vi "002_FlowChart.vi"(11 "Queue Ref":T1={"UI"=refnum, "Message"=refnum, "Data"=refnum, "Caller"=refnum, "Name"="000 Common", "Data Path"=path "", "Class Path"=path "", "SubPanel"=refnum, "Project Name"="", "MNT"="", "Title"="", "Data Source"=refnum, "Queue List"={}, "VI"=refnum, "UE"=refnum}) -> ()   [LabVIEW 2020]
doc: "0014_XAJD_1500W-Flow Chart"
uses:
  Alin/QMH/000 Module Data Type.ctl
  Alin/QMH/Queue Message.ctl
  <vilib>/Utility/miscctls.llb/LVPoint32TypeDef.ctl
  a1345304-ed38-41b0-8c79-7ce0969963d6.vi
  <vilib>/Utility/file.llb/Read Delimited Spreadsheet (string).vi
  <vilib>/Utility/file.llb/Write Delimited Spreadsheet (string).vi
panel:
  out "QN":i32
  in  "ShowLable":bool
  in  "Chart Select":u16(ring) items=["0014_XAJD_1500W.vi", "0014_XAJD_1500W_1.vi"]
  in  "Panel Show":bool
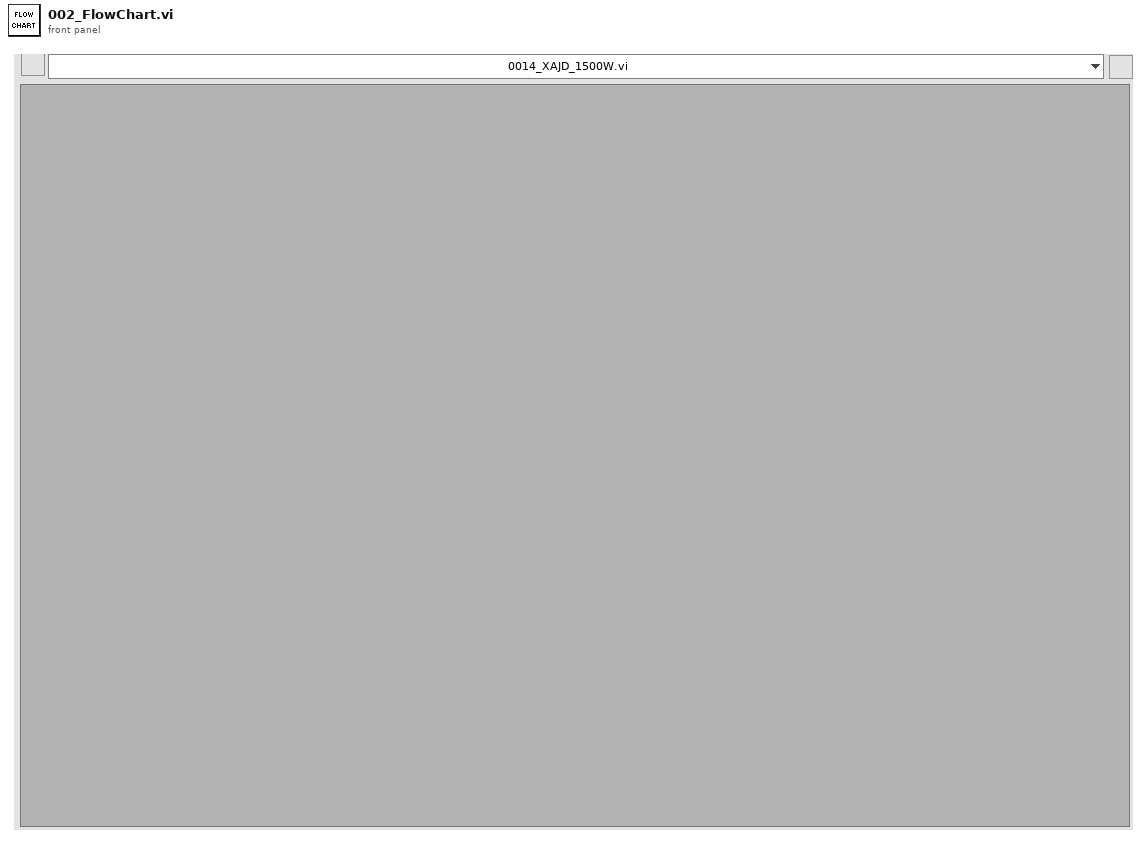
[diagram p1: front panel]
types:
  T1 = typedef "000 Module Data Type.ctl" = cluster{"UI":refnum<queue>, "Message":refnum<queue>, "Data":refnum<queue>, "Caller":refnum<queue>, "Name":string, "Data Path":path, "Class Path":path, "SubPanel":refnum<vi>, "Project Name":string, "MNT":string, "Title":string, "Data Source":refnum<queue>, "Queue List":map{string, refnum<queue>}, "VI":refnum<vi>, "UE":refnum<user-event>}
  T2 = enum32{"Invalid", "Standard", "Closed", "Hidden", "Minimized", "Maximized"}
  T3 = cluster{"Queue Ref":T1, "Flow Chart":refnum<vi>, "Controls":refnum<vi>[], "Delay":cluster{"Count Time(ms)":u32, "Delay Time(ms)":u32, "Next":string}}
  T4 = typedef "SDQ Data Type.ctl" = cluster{"CAN Length":string, "CAN Name":string, "CAN ID":string, "CAN Type":string, "Test Item":string, "Byte Order":string, "Instruction":string, "Control Type":string, "Group":string, "Offset":dbl, "Coefficient":dbl, "Write Enable":bool, "Lable Type":string, "Key?":string, "Set Value":string, "Upper":dbl, "Lower":dbl, "Unit":string, "Formula":string, "Test Item Type":string, "Length":i32, "Address":string, "Name":string, "Identifier":string, "Data Type":string, "Enumerate?":string, "Enumerate List":string, "Data":string, "Source":string}
  T5 = enum8{"Enabled", "Disabled", "Disabled and Grayed Out"}
  T6 = typedef "eventvkey.ctl" = enum16{"ASCII", "Enter", "Return", "Shift", "Ctrl", "Alt", "Cmd", "Opt", "Caps", "NumLock", "Clear", "Break", "Up", "Down", "Left", "Right", "Insert", "Delete", "Home", "End", "PageUp", "PageDown", "Escape", "Help", "Pause", "ScrollLock", "F1", "F2", "F3", "F4", "F5", "F6", "F7", "F8", "F9", "F10", "F11", "F12", "F13", "F14", "F15", "F16", "F17", "F18", "F19", "F20", "F21", "F22", "F23", "F24", "Play", "VolumeUp", "VolumeDown", "Mute", "Two Byte Char"}
  T7 = cluster{"Shift":bool, "Ctrl":bool, "Alt":bool, "Cmd":bool, "Opt":bool}
  T8 = typedef "LVPoint32TypeDef.ctl" = cluster{"Horizontal":i32, "Vertical":i32}
  T9 = cluster{"Queue List":map{string, refnum<queue>}, "SubPanel":refnum<vi>, "Active Panel":string, "Queue Ref":T1, "Project Name":string, "FlowChart":refnum<vi>, "Controls":refnum<vi>[]}
  T10 = typedef "LVBoundsTypeDef.ctl" = cluster{"Width":u32, "Height":u32}
  T11 = typedef "LVPointTypeDef.ctl" = cluster{"Horizontal":i16, "Vertical":i16}
  T12 = typedef "LVPositionTypeDef.ctl" = cluster{"Left":i32, "Top":i32}
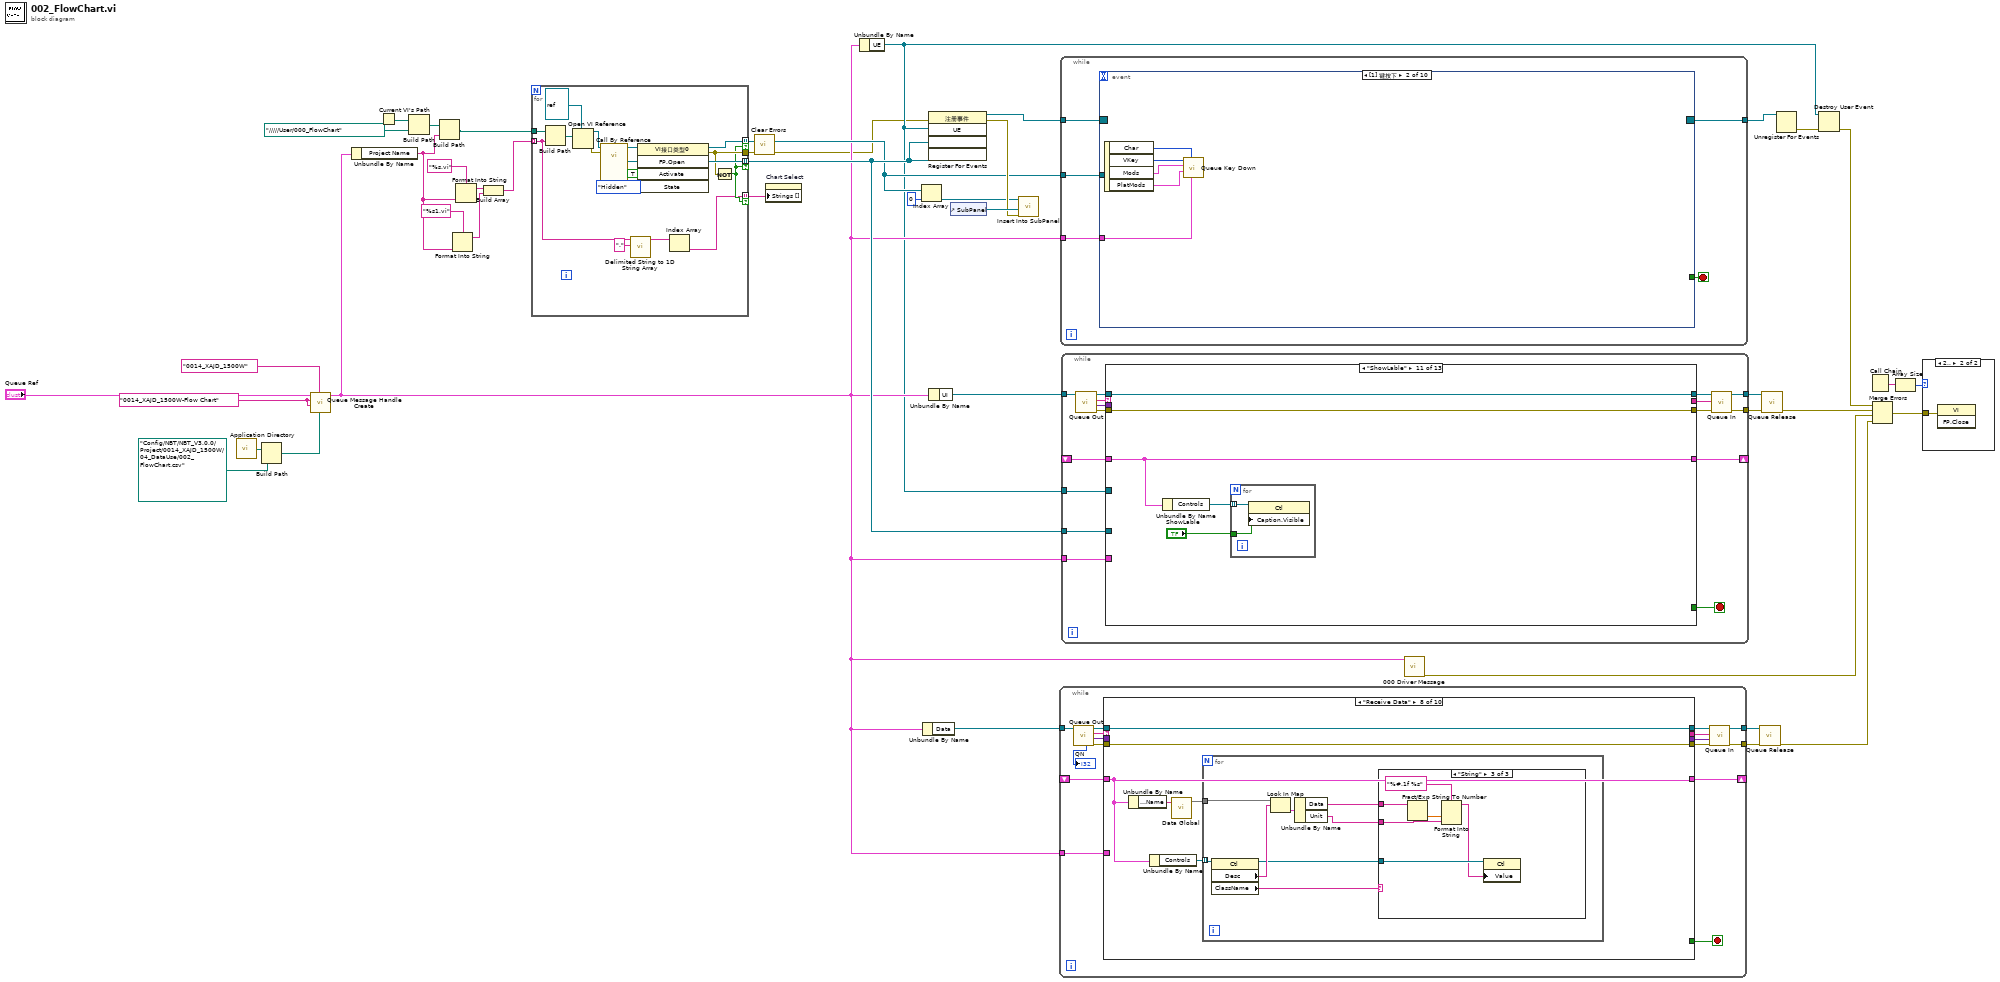
[diagram p0: block diagram]
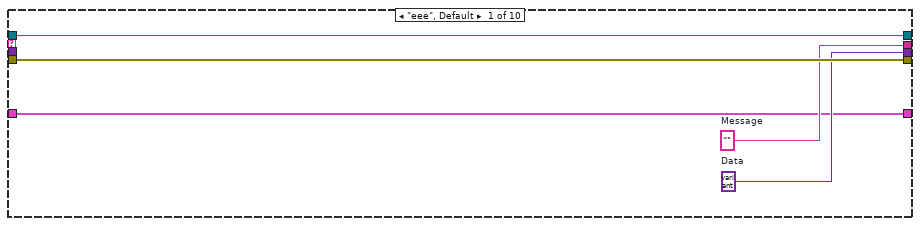
[diagram p2: hidden frame]
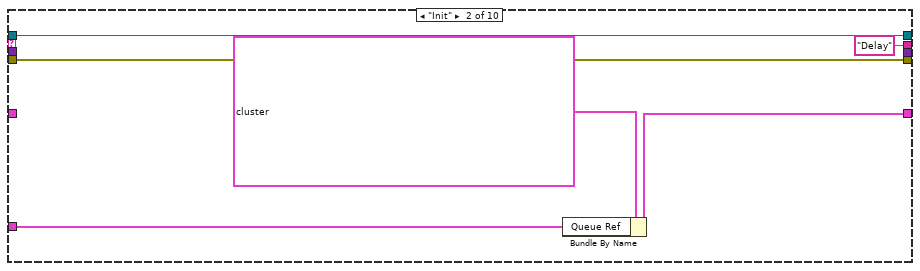
[diagram p3: hidden frame]
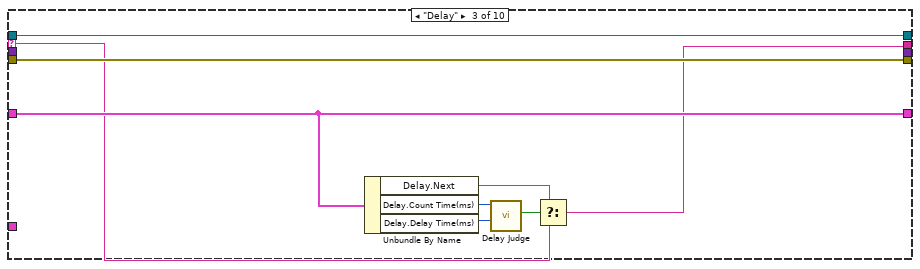
[diagram p4: hidden frame]
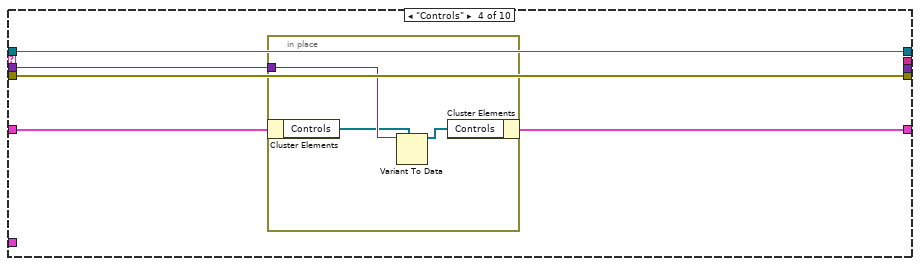
[diagram p5: hidden frame]
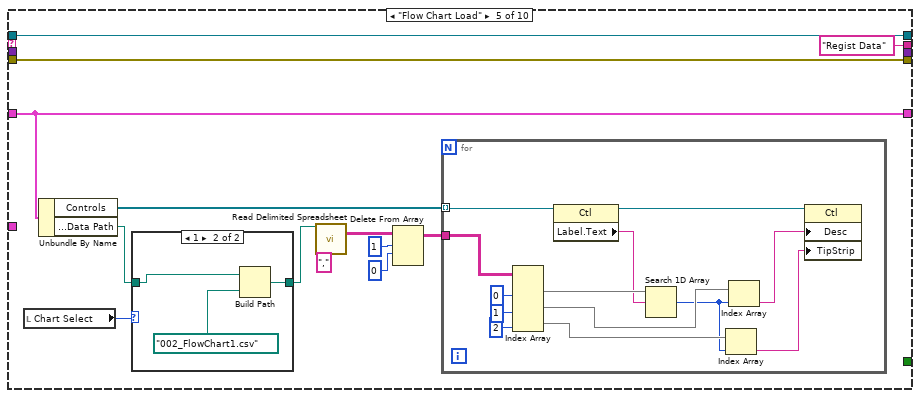
[diagram p6: hidden frame]
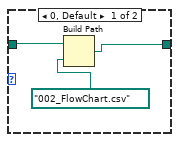
[diagram p7: hidden frame]
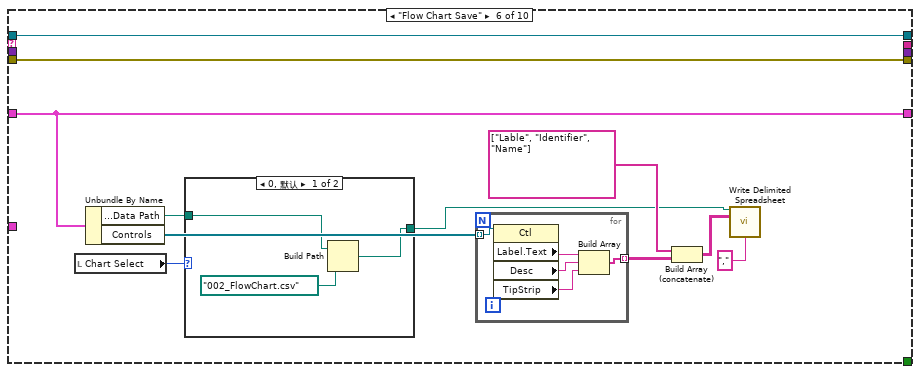
[diagram p8: hidden frame]
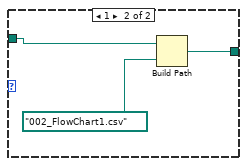
[diagram p9: hidden frame]
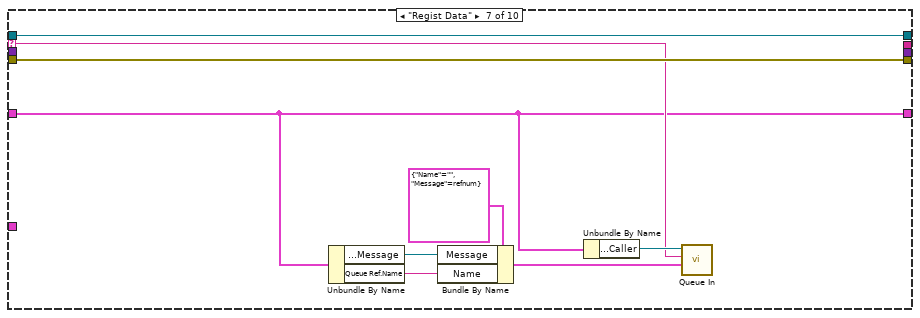
[diagram p10: hidden frame]
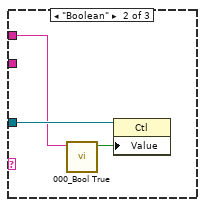
[diagram p12: hidden frame]
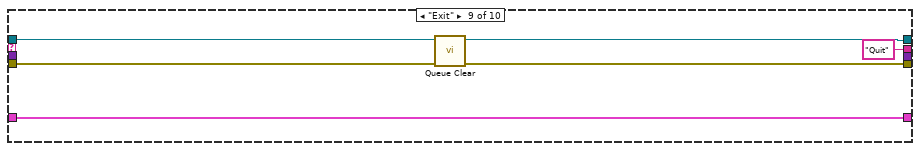
[diagram p13: hidden frame]
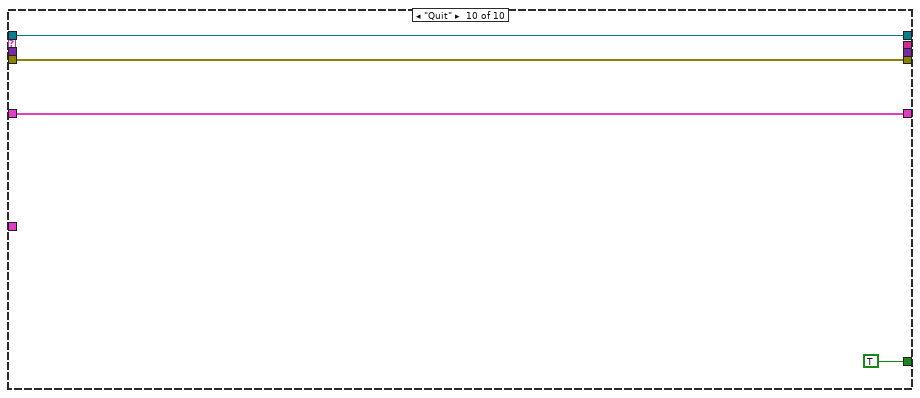
[diagram p14: hidden frame]
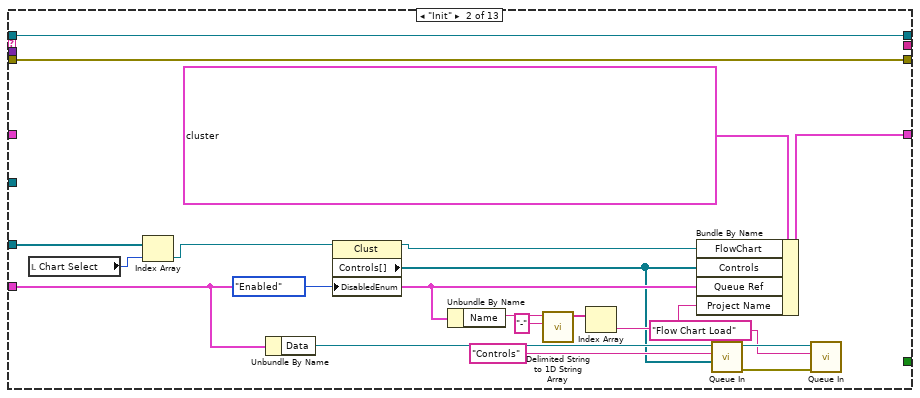
[diagram p17: hidden frame]
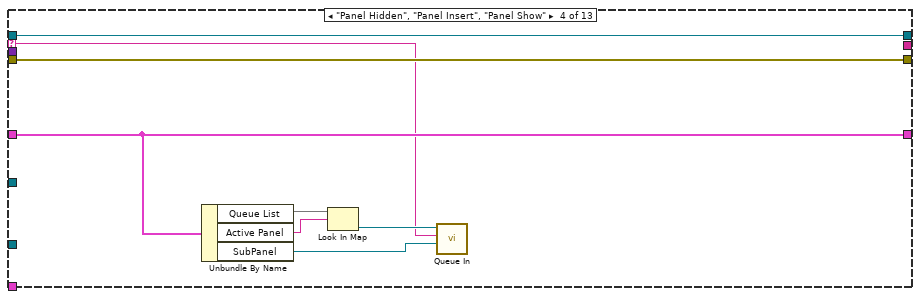
[diagram p19: hidden frame]
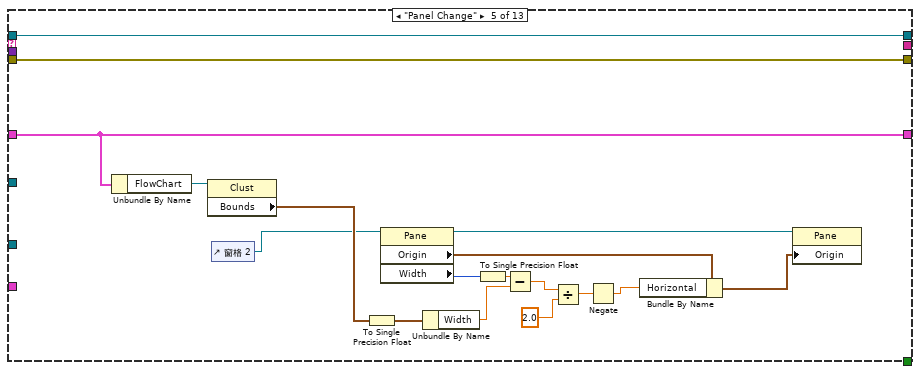
[diagram p20: hidden frame]
diagram:
  w6 = "0014_XAJD_1500W-Flow Chart" ("Name")
  n1 = call <vilib>:"Application Directory.vi"() -> ("Application Directory"=w9:path)
  n2 = Build Path(base path=w9, name or relative path=path "Config/NBT/NBT_V3.0.0/Project/0014_XAJD_1500W/04_DataUse/002_FlowChart.csv" ("名称或相对路径")) -> (appended path=w7:path)
  n3 = call "Queue Message Handle Create.vi"("Data Path"=w7, "Project Name"="0014_XAJD_1500W" ("Name"), "Name"=w6, "Title"=w6, "Queue Ref In"="Queue Ref") -> ("Queue Ref Out"=w3:T1)  [unwired: 5 in, 1 out]
  n4 = Unbundle By Name(w3) -> ("Project Name"=w12:string)
  n5 = Current VI's Path() -> (path=w27:path)
  n6 = Build Path(base path=w27, name or relative path=path "../../../../../User/000_FlowChart" ("名称或相对路径")) -> (appended path=w25:path)
  n7 = Build Path(base path=w25, name or relative path=w12) -> (appended path=w19:path)
  n8 = Format Into String(format string="%s1.vi" ("格式字符串"), w12) -> (resulting string=w11:string)  [unwired: 2 in, 1 out]
  n9 = Format Into String(format string="%s.vi" ("格式字符串"), w12) -> (resulting string=w17:string)  [unwired: 2 in, 1 out]
  n10 = Build Array(w17, w11) -> (w10:string[])
  n11 = for {
    tunnel: [w49] -> w22
    tunnel: [w53] -> w14 mode=indexing if=w48
    tunnel: [w52] -> w21 mode=indexing if=w48
    tunnel: w19 -> [w51]
    tunnel: w10 -> [w47] mode=indexing
    tunnel: [w44] -> w4 mode=indexing if=w48
    n12 = Build Path(base path=w51, name or relative path=w47) -> (appended path=w50:path)
    n13 = Open VI Reference(type specifier VI Refnum (for type only)=refnum<vi> refnum ("类型说明符VI引用句柄（仅用于类型）"), vi path=w50) -> (vi reference=w58:refnum<vi>, error out=w59:errorcluster)  [unwired: 4 in]
    n14 = call-by-ref "?"(reference=w58, error in=w59) -> (reference out=w56:refnum<vi>, "Cluster"=w52:refnum<vi>)  [unwired: 11 in, 1 out]
    n15 = call <vilib>:"Delimited String to 1D String Array.vi"("delimiter"=".", "delimited string"=w47) -> ("string array"=w45:string[])  [unwired: 9 in]
    n16 = invoke class="VI接口类型0" method="FP.Open"(reference=w56, "Activate"=TRUE ("激活？"), "State"=T2."Hidden" ("状态")) -> (reference out=w53:refnum<vi>, error out=w49:errorcluster)  [unwired: 2 in, 3 out]
    n17 = Index Array(array=w45) -> (element=w44:string)  [unwired: 1 in]
    n18 = Not(x=w49) -> (.not. x?=w48:bool)
  }
  n19 = call <vilib>:"Clear Errors.vi"("error in (no error)"=w22) -> ("error out"=w1:errorcluster)  [unwired: 5 in, 1 out]
  n20 = property on="Chart Select" class="Ring (严格)"("Strings []"=w4) -> ()  [unwired: 2 in, 2 out]
  n21 = Unbundle By Name(w3) -> ("UE"=w2:refnum<user-event>)
  n22 = Index Array(array=w14, index=0 ("索引")) -> (element=w16:refnum<vi>)
  n23 = Unbundle By Name(w3) -> ("Data"=w41:refnum<queue>)
  n24 = register-events(error in=w1, w2, w21, w21) -> (reference out=w28:refnum<event-registration>, error out=w23:errorcluster)  [unwired: 1 in]
  n25 = Unbundle By Name(w3) -> ("UI"=w33:refnum<queue>)
  n26 = control-ref of="SubPanel"() -> (w24:refnum<vi>)
  n27 = call "Insert Into SubPanel.vi"("error in (no error)"=w23, "SubPanel Ref"=w24, "VI Ref In"=w16) -> ()  [unwired: 8 in, 1 out]
  n28 = while {
    tunnel: w41 -> [w71]
    tunnel: [w68] -> w39
    tunnel: [w67] -> w40
    shift-right: [w63] -> _
    shift-left: _ -> [w62]
    tunnel: w3 -> [w61]
    stop <- w75 stop-if-true
    n29 = call "Queue Out.vi"("Queue In"=w71) -> ("error out"=w74:errorcluster, "Data"=w72:variant, "Message"=w73:string, "Queue Out"=w70:refnum<queue>, "Queue NUmber"=→"QN":i32)  [unwired: 6 in]
    n30 = case shown="\"Receive Data\"" w73 {
      selector: w73 -> [_ _ w88 _ _ _ w162 _ _ _]
      tunnel: w70 -> [w80 w86 w95 w100 w116 w146 w166 w172 w194 w198]
      tunnel: w74 -> [w79 w85 w94 w99 w115 w145 w165 w171 w192 w199]
      tunnel: [w80 w86 w95 w100 w116 w146 w166 w172 w193 w198] -> w69
      tunnel: [w79 w85 w94 w99 w115 w145 w165 w171 w191 w199] -> w66
      tunnel: [w78 "Delay" ("Message") w87 _ "Regist Data" ("Message") _ _ _ "Quit" _] -> w65
      tunnel: [_ _ _ _ _ _ _ _ _ TRUE] -> w75
      tunnel: [w77 _ _ _ _ _ _ _ _ _] -> w64
      tunnel: w72 -> [_ _ _ w96 _ _ _ _ _ _]
      tunnel: [w76 w83 w89 w97 w114 w144 w159 w168 w190 w196] -> w63
      tunnel: w62 -> [w76 _ w89 w98 w114 w144 w159 w168 w190 w196]
      tunnel: w61 -> [_ w82 _ _ _ _ _ _ _ _]
      frame "eee", Default {
        w77 = variant  # Data
        w78 = ""  # Message
      }
      frame "Init" {
        n31 = Bundle By Name(cluster=T3 {"Queue Ref"={"UI"=refnum, "Message"=refnum, "Data"=refnum, "Caller"=refnum, "Name"="", "Data Path"=path "", "Class Path"=path "", "SubPanel"=refnum, "Project Name"="", "MNT"="", "Title"="", "Data Source"=refnum, "Queue List"={}, "VI"=refnum, "UE"=refnum}, "Flow Chart"=refnum, "Controls"=[], "Delay"={"Count Time(ms)"=250, "Delay Time(ms)"=250, "Next"="Receive Data,Delay"}}, "Queue Ref"=w82) -> (w83:T3)
      }
      frame "Delay" {
        n32 = Unbundle By Name(w89) -> ("Delay.Next"=w93:string, "Delay.Count Time(ms)"=w90:u32, "Delay.Delay Time(ms)"=w91:u32)
        n33 = call "Delay Judge.vi"("Delay Time(ms)"=w91, "Count Time(ms)"=w90) -> ("Time Out?"=w92:bool)  [unwired: 5 in, 4 out]
        n34 = Select(t=w93, s=w92, f=w88) -> (s? t:f=w87:string)
      }
      frame "Controls" {
        n35 = in-place {
          in-place-border: w96 -> [w103]
          n36 = in-place-cluster #1(w98) -> ("Controls"=w102:refnum<vi>[])
          n37 = Variant To Data(type=w102, Variant=w103) -> (data=w101:refnum<vi>[])  [unwired: 1 in, 1 out]
          n38 = in-place-cluster #1("Controls"=w101) -> (w97:T3)
        }
      }
      frame "Flow Chart Load" {
        n39 = local read "Chart Select"() -> (w106:u16)
        n40 = Unbundle By Name(w114) -> ("Controls"=w113:refnum<vi>[], "Queue Ref.Data Path"=w105:path)
        n41 = case shown="1" w106 {
          tunnel: w105 -> [w119 w120]
          tunnel: [w117 w121] -> w104
          frame 0, Default {
            n42 = Build Path(base path=w119, name or relative path=path "002_FlowChart.csv" ("名称或相对路径")) -> (appended path=w117:path)
          }
          frame 1 {
            n43 = Build Path(base path=w120, name or relative path=path "002_FlowChart1.csv" ("名称或相对路径")) -> (appended path=w121:path)
          }
        }
        n44 = call-poly <vilib>:"Read Delimited Spreadsheet.vi"("file path (dialog if empty)"=w104, "delimiter (\\t)"="," ("delimiter (\\t)")) -> ("all rows"=w111:string[][])  [unwired: 8 in, 5 out]
        n45 = Delete From Array(array=w111, length=1 ("长度"), index (row)=0 ("索引 (行)")) -> (array with subset deleted=w108:string[][])  [unwired: 1 in, 1 out]
        n46 = for {
          tunnel: w113 -> [w135] mode=indexing
          tunnel: w108 -> [w134]
          n47 = Index Array(array=w134, index (col) #1=0 ("禁用的索引 (列)"), index (col) #2=1 ("索引 (列)"), index (col) #3=2 ("索引 (列)")) -> (element #1=w131:string[], element #2=w129:string[], element #3=w125:string[])  [unwired: 3 in]
          n48 = property class="Ctl"(reference=w135) -> (reference out=w128:refnum<vi>, "Label.Text"=w130:string)  [unwired: 1 in, 1 out]
          n49 = Search 1D Array(1D array=w131, element=w130) -> (index of element=w124:i32)  [unwired: 1 in]
          n50 = Index Array(array=w125, index=w124) -> (element=w123:string)
          n51 = Index Array(array=w129, index=w124) -> (element=w127:string)
          n52 = property class="Ctl"(reference=w128, "Desc"=w127, "TipStrip"=w123) -> ()  [unwired: 1 in, 2 out]
        }
      }
      frame "Flow Chart Save" {
        n53 = local read "Chart Select"() -> (w138:u16)
        n54 = Unbundle By Name(w144) -> ("Queue Ref.Data Path"=w137:path, "Controls"=w143:refnum<vi>[])
        n55 = case shown="0, 默认" w138 {
          tunnel: w137 -> [w148 w152]
          tunnel: [w149 w150] -> w136
          frame 0, Default {
            n56 = Build Path(base path=w148, name or relative path=path "002_FlowChart.csv" ("名称或相对路径")) -> (appended path=w149:path)
          }
          frame 1 {
            n57 = Build Path(base path=w152, name or relative path=path "002_FlowChart1.csv" ("名称或相对路径")) -> (appended path=w150:path)
          }
        }
        n58 = for {
          tunnel: w143 -> [w157] mode=indexing
          tunnel: [w154] -> w141 mode=indexing
          n59 = property class="Ctl"(reference=w157) -> ("Label.Text"=w156:string, "Desc"=w155:string, "TipStrip"=w153:string)  [unwired: 1 in, 2 out]
          n60 = Build Array(w156, w155, w153) -> (w154:string[])
        }
        n61 = Build Array (concatenate)(string[] ["Lable", "Identifier", "Name"], w141) -> (w140:string[][])
        n62 = call-poly <vilib>:"Write Delimited Spreadsheet.vi"("file path (dialog if empty)"=w136, "2D data"=w140, "delimiter (\\t)"="," ("delimiter (\\t)")) -> ()  [unwired: 11 in, 2 out]
      }
      frame "Regist Data" {
        n63 = Unbundle By Name(w159) -> ("Queue Ref.Message"=w160:refnum<queue>, "Queue Ref.Name"=w158:string)
        n64 = Bundle By Name(cluster=cluster{"Name":string, "Message":refnum<queue>} {"Name"="", "Message"=refnum} ("输出簇"), "Message"=w160, "Name"=w158) -> (w161:cluster{"Name":string, "Message":refnum<queue>})
        n65 = Unbundle By Name(w159) -> ("Queue Ref.Caller"=w163:refnum<queue>)
        n66 = call "Queue In.vi"("Data"=w161, "Message"=w162, "Queue In"=w163) -> ()  [unwired: 7 in, 2 out]
      }
      frame "Receive Data" {
        n67 = Unbundle By Name(w168) -> ("Queue Ref.Name"=w169:string)
        n68 = Unbundle By Name(w168) -> ("Controls"=w170:refnum<vi>[])
        n69 = call "Data Global.vi"("Name"=w169) -> ("Data Out"=w167:map{string, T4})  [unwired: 7 in, 3 out]
        n70 = for {
          tunnel: w170 -> [w180] mode=indexing
          tunnel: w167 -> [w179]
          n71 = property class="Ctl"(reference=w180) -> (reference out=w175:refnum<vi>, "Desc"=w178:string, "ClassName"=w176:string)  [unwired: 1 in, 1 out]
          n72 = Look In Map(map=w179, key=w178) -> (value=w177:T4)  [unwired: 1 in, 1 out]
          n73 = Unbundle By Name(w177) -> ("Data"=w174:string, "Unit"=w173:string)
          n74 = case shown="\"String\"" w176 {
            tunnel: w175 -> [_ w183 w189]
            tunnel: w174 -> [_ w182 w186]
            tunnel: w173 -> [_ _ w184]
            frame "eee", Default {
            }
            frame "Boolean" {
              n75 = call "000_Bool True.vi"("Bool String"=w182) -> ("True"=w181:bool)  [unwired: 8 in, 2 out]
              n76 = property class="Ctl"(reference=w183, "Value"=w181) -> ()  [unwired: 1 in, 2 out]
            }
            frame "String" {
              n77 = Fract/Exp String To Number(string=w186) -> (number=w185:dbl)  [unwired: 3 in, 1 out]
              n78 = Format Into String(format string="%#.1f %s" ("格式字符串"), w185, w184) -> (resulting string=w187:string)  [unwired: 2 in, 1 out]
              n79 = property class="Ctl"(reference=w189, "Value"=w187) -> ()  [unwired: 1 in, 2 out]
            }
          }
        }
      }
      frame "Exit" {
        n80 = call "Queue Clear.vi"("error in (no error)"=w192, "Queue In"=w194) -> ("error out"=w191:errorcluster, "Queue Out"=w193:refnum<queue>)  [unwired: 8 in]
      }
      frame "Quit" {
      }
    }
    n81 = call "Queue In.vi"("error in (no error)"=w66, "Data"=w64, "Message"=w65, "Queue In"=w69) -> ("error out"=w67:errorcluster, "Queue Out"=w68:refnum<queue>)  [unwired: 6 in]
  }
  n82 = while {
    tunnel: w28 -> [w204]
    tunnel: [w202] -> w29
    tunnel: w3 -> [w201]
    tunnel: w14 -> [w200]
    stop <- w203 stop-if-true
    n83 = event shown="[1] 键按下" {
      selector: w204 -> [_ _ _ _ _ _ _ _ _ _]
      dyn-events: [_ _ _ _ _ _ _ _ _ _] -> w202
      timeout: _ -> [_ _ _ _ _ _ _ _ _ _]
      tunnel: [_ _ _ _ _ w243 _ _ _ _] -> w203
      tunnel: w201 -> [_ w208 w212 w218 w223 _ w247 w256 w264 w268]
      tunnel: w200 -> [_ _ _ _ _ _ _ w259 _ _]
      event Timeout {
        n84 = event-data() -> ()  [unwired: 1 in, 1 out]
      }
      event Key Down {
        n85 = event-data() -> ("Char"=w209:i16, "VKey"=w207:T6, "Mods"=w206:cluster{"Num Pad":bool, "Menu Key":bool}, "PlatMods"=w205:T7)  [unwired: 1 in]
        n86 = call "Queue Key Down.vi"("Queue Ref Out"=w208, "C"=w209, "Platform Key"=w205, "Group Key"=w206, "V Key"=w207) -> ()  [unwired: 6 in, 1 out]
      }
      event Panel Resize {
        n87 = event-data() -> ()  [unwired: 1 in, 1 out]
        n88 = Unbundle By Name(w212) -> ("Message"=w211:refnum<queue>)
        n89 = call "Queue In.vi"("Message"="Panel Change", "Queue In"=w211) -> ()  [unwired: 8 in, 2 out]
      }
      event Value Change {
        n90 = event-data() -> ("NewVal"=w217:variant, "OldVal"=w216:variant)  [unwired: 1 in]
        n91 = Unbundle By Name(w218) -> ("UI"=w215:refnum<queue>)
        n92 = call "FlowChart String Analize.vi"("Old Value"=w216, "New Value"=w217) -> ("Data"=w214:cluster{"Index":i32, "Data":variant})  [unwired: 7 in, 2 out]
        n93 = call "Queue In.vi"("Data"=w214, "Message"="Write Prepare", "Queue In"=w215) -> ()  [unwired: 7 in, 2 out]
      }
      event Mouse Down {
        n94 = event-data() -> ("CtlRef"=w220:refnum<vi>, "PlatMods.Shift"=w221:bool, "Coords"=w219:T8, "PlatMods.Alt"=w224:bool, "Mods.Double Click"=w225:bool)  [unwired: 1 in]
        n95 = Unbundle By Name(w223) -> ("UI"=w222:refnum<queue>)
        n96 = case shown="真" w225 {
          tunnel: w224 -> [_ w230]
          tunnel: w222 -> [_ w229]
          tunnel: w221 -> [_ w228]
          tunnel: w220 -> [_ w227]
          tunnel: w219 -> [_ w226]
          frame False {
          }
          frame True {
            n97 = case shown="真" w230 {
              tunnel: w229 -> [_ w242]
              tunnel: w228 -> [w232 _]
              tunnel: w227 -> [w231 _]
              tunnel: w226 -> [_ w240]
              frame False {
                n98 = case shown="真" w232 {
                  tunnel: w231 -> [_ w233]
                  frame False {
                  }
                  frame True {
                    n99 = property class="Clust"(reference=w233) -> (reference out=w235:refnum<vi>, "DisabledEnum"=w234:T5)  [unwired: 1 in, 1 out]
                    n100 = case shown="\"Enabled\", 默认" w234 {
                      tunnel: [T5."Disabled and Grayed Out" ("禁用") T5."Disabled and Grayed Out" ("禁用") T5."Enabled" ("禁用")] -> w236
                      frame "Enabled", Default {
                      }
                      frame "Disabled" {
                      }
                      frame "Disabled and Grayed Out" {
                      }
                    }
                    n101 = property class="Clust"(reference=w235, "DisabledEnum"=w236) -> ()  [unwired: 1 in, 2 out]
                  }
                }
              }
              frame True {
                n102 = call "Queue In.vi"("Data"=w240, "Message"="Show Data Source", "Queue In"=w242) -> ()  [unwired: 7 in, 2 out]
              }
            }
          }
        }
      }
      event User Event {
        n103 = event-data() -> ("Message"=w245:string)  [unwired: 1 in]
        n104 = Equal?(x=w245, y="Exit") -> (x = y?=w243:bool)
      }
      event Panel Close? {
        n105 = event-data() -> ()  [unwired: 1 in, 1 out]
        n106 = Unbundle By Name(w247) -> ("Message"=w246:refnum<queue>)
        n107 = Call Chain() -> (call chain=w250:string[])
        n108 = Array Size(array=w250) -> (size(s)=w249:i32)
        n109 = case shown="0, 默认" w249 {
          tunnel: ["Exit Prepare" ("Message") "Panel Hidden" ("Message")] -> w248
          frame 0, Default {
          }
          frame 2.. {
          }
        }
        n110 = call "Queue In.vi"("Message"=w248, "Queue In"=w246) -> ()  [unwired: 8 in, 2 out]
        n111 = event-data("Discard?"=TRUE ("放弃？")) -> ()  [unwired: 1 in, 1 out]
      }
      event "Chart Select": Value Change {
        n112 = event-data() -> ()  [unwired: 1 in, 1 out]
        n113 = Unbundle By Name(w256) -> ("UI"=w255:refnum<queue>)
        n114 = call "Queue In.vi"("Message"="Init", "Queue In"=w255) -> ()  [unwired: 8 in, 2 out]
        n115 = control-ref of="SubPanel"() -> (w260:refnum<vi>)
        n116 = Index Array(array=w259, index="Chart Select") -> (element=w257:refnum<vi>)
        n117 = call "Insert Into SubPanel.vi"("SubPanel Ref"=w260, "VI Ref In"=w257) -> ()  [unwired: 9 in, 1 out]
      }
      event "Panel Show": Value Change {
        n118 = event-data() -> ("CtlRef"=w262:refnum<vi>)  [unwired: 1 in]
        n119 = Unbundle By Name(w264) -> ("Message"=w263:refnum<queue>)
        n120 = property class="Bool"(reference=w262) -> ("Label.Text"=w261:string)  [unwired: 1 in, 2 out]
        n121 = call "Queue In.vi"("Message"=w261, "Queue In"=w263) -> ()  [unwired: 8 in, 2 out]
      }
      event "ShowLable": Value Change {
        n122 = event-data() -> ("CtlRef"=w266:refnum<vi>)  [unwired: 1 in]
        n123 = Unbundle By Name(w268) -> ("UI"=w267:refnum<queue>)
        n124 = property class="Bool (严格)"(reference=w266) -> ("Label.Text"=w265:string)  [unwired: 1 in, 2 out]
        n125 = call "Queue In.vi"("Message"=w265, "Queue In"=w267) -> ()  [unwired: 8 in, 2 out]
      }
    }
  }
  n126 = while {
    tunnel: w33 -> [w279]
    tunnel: [w276] -> w31
    tunnel: [w275] -> w32
    tunnel: w2 -> [w283]
    tunnel: w3 -> [w272]
    shift-right: [w271] -> _
    shift-left: _ -> [w270]
    tunnel: w21 -> [w269]
    stop <- w284 stop-if-true
    n127 = call "Queue Out.vi"("Queue In"=w279) -> ("error out"=w282:errorcluster, "Data"=w280:variant, "Message"=w281:string, "Queue Out"=w278:refnum<queue>)  [unwired: 6 in, 1 out]
    n128 = case shown="\"ShowLable\"" w281 {
      selector: w281 -> [_ _ _ w313 _ _ w346 _ _ _ _ w433 _]
      tunnel: w278 -> [w287 w307 w310 w318 w335 w340 w350 w353 w363 w409 w428 w440 w447]
      tunnel: w282 -> [w286 w306 w309 w317 w334 w339 w349 w352 w362 w408 w427 w438 w448]
      tunnel: [w287 w307 w310 w318 w335 w340 w350 w353 w363 w409 w428 w439 w447] -> w277
      tunnel: [w286 w306 w309 w317 w334 w339 w349 w352 w362 w408 w427 w437 w448] -> w274
      tunnel: [_ _ _ _ _ _ _ _ _ _ _ "Quit" _] -> w273
      tunnel: [_ _ _ _ _ _ _ _ _ _ _ _ TRUE] -> w284
      tunnel: w283 -> [_ _ _ _ _ _ _ _ _ _ _ _ _]
      tunnel: w280 -> [_ _ _ _ _ w336 _ _ w360 w406 _ _ _]
      tunnel: w272 -> [_ w294 _ _ _ _ w348 _ _ _ _ _ _]
      tunnel: [w285 w304 w308 w316 w333 w337 w345 w351 w354 w405 w426 w432 w445] -> w271
      tunnel: w270 -> [w285 _ w308 w316 w333 w338 w345 w351 w355 w405 w426 w432 w445]
      tunnel: w269 -> [_ w297 _ _ _ _ _ _ _ _ _ _ _]
      frame "eee", Default {
      }
      frame "Init" {
        n129 = local read "Chart Select"() -> (w296:u16)
        n130 = Index Array(array=w297, index=w296) -> (element=w295:refnum<vi>)
        n131 = Unbundle By Name(w294) -> ("Data"=w293:refnum<queue>)
        n132 = property class="Clust"(reference=w295, "DisabledEnum"=T5."Enabled" ("禁用")) -> (reference out=w298:refnum<vi>, "Controls[]"=w291:refnum<vi>[])  [unwired: 1 in, 1 out]
        n133 = Unbundle By Name(w294) -> ("Name"=w303:string)
        n134 = call <vilib>:"Delimited String to 1D String Array.vi"("delimiter"="-", "delimited string"=w303) -> ("string array"=w301:string[])  [unwired: 9 in]
        n135 = Index Array(array=w301) -> (element=w300:string)  [unwired: 1 in]
        n136 = Bundle By Name(cluster=T9 {"Queue List"={}, "SubPanel"=refnum, "Active Panel"="", "Queue Ref"={"UI"=refnum, "Message"=refnum, "Data"=refnum, "Caller"=refnum, "Name"="", "Data Path"=path "", "Class Path"=path "", "SubPanel"=refnum, "Project Name"="", "MNT"="", "Title"="", "Data Source"=refnum, "Queue List"={}, "VI"=refnum, "UE"=refnum}, "Project Name"="", "FlowChart"=refnum, "Controls"=[]}, "FlowChart"=w298, "Controls"=w291, "Queue Ref"=w294, "Project Name"=w300) -> (w304:T9)
        n137 = call "Queue In.vi"("Data"=w291, "Message"="Controls", "Queue In"=w293) -> ("error out"=w290:errorcluster, "Queue Out"=w289:refnum<queue>)  [unwired: 7 in]
        n138 = call "Queue In.vi"("error in (no error)"=w290, "Message"="Flow Chart Load", "Queue In"=w289) -> ()  [unwired: 7 in, 2 out]
      }
      frame "====System====" {
      }
      frame "Panel Hidden", "Panel Insert", "Panel Show" {
        n139 = Unbundle By Name(w316) -> ("Queue List"=w315:map{string, refnum<queue>}, "Active Panel"=w312:string, "SubPanel"=w311:refnum<vi>)
        n140 = Look In Map(map=w315, key=w312) -> (value=w314:refnum<queue>)  [unwired: 1 in, 1 out]
        n141 = call "Queue In.vi"("Data"=w311, "Message"=w313, "Queue In"=w314) -> ()  [unwired: 7 in, 2 out]
      }
      frame "Panel Change" {
        n142 = Unbundle By Name(w333) -> ("FlowChart"=w331:refnum<vi>)
        n143 = property class="Clust"(reference=w331) -> ("Bounds"=w332:T10)  [unwired: 1 in, 2 out]
        n144 = control-ref of="窗格 2"() -> (w319:refnum<vi>)
        n145 = To Single Precision Float(number=w332) -> (single precision float=w324:cluster{"Width":sgl, "Height":sgl})
        n146 = property class="Pane"(reference=w319) -> (reference out=w326:refnum<vi>, "Origin"=w322:T11, "Width"=w330:u32)  [unwired: 1 in, 1 out]
        n147 = Unbundle By Name(w324) -> ("Width"=w323:sgl)
        n148 = To Single Precision Float(number=w330) -> (single precision float=w325:sgl)
        n149 = Subtract(x=w325, y=w323) -> (x-y=w329:sgl)
        n150 = Divide(x=w329, y=sgl 2.0) -> (x/y=w327:sgl)
        n151 = Negate(x=w327) -> (-x=w321:sgl)
        n152 = Bundle By Name(cluster=w322, "Horizontal"=w321) -> (w320:T11)
        n153 = property class="Pane"(reference=w326, "Origin"=w320) -> ()  [unwired: 1 in, 2 out]
      }
      frame "Send Client Refer" {
        n154 = in-place {
          in-place-border: w336 -> [w342]
          n155 = in-place-cluster #2(w338) -> ("Queue List"=w341:map{string, refnum<queue>})
          n156 = Variant To Data(type=w341, Variant=w342) -> (data=w343:map{string, refnum<queue>})  [unwired: 1 in, 1 out]
          n157 = in-place-cluster #2("Queue List"=w343) -> (w337:T9)
        }
      }
      frame "Client Delete", "Client Launch" {
        n158 = Unbundle By Name(w348) -> ("Message"=w347:refnum<queue>)
        n159 = Unbundle By Name(w345) -> ("Active Panel"=w344:string)
        n160 = call "Queue In.vi"("Data"=w344, "Message"=w346, "Queue In"=w347) -> ()  [unwired: 7 in, 2 out]
      }
      frame "====User====" {
      }
      frame "Show Data Source" {
        n161 = Unbundle By Name(w355) -> ("FlowChart"=w359:refnum<vi>)
        n162 = Variant To Data(type=T8 {"Horizontal"=0, "Vertical"=0} ("坐标"), Variant=w360) -> (data=w356:T8)  [unwired: 1 in, 1 out]
        n163 = property class="Clust"(reference=w359) -> ("DisabledEnum"=w358:T5, "Controls[]"=w357:refnum<vi>[])  [unwired: 1 in, 2 out]
        n164 = case shown="\"Disabled and Grayed Out\"" w358 {
          tunnel: w357 -> [_ w368]
          tunnel: w356 -> [_ w367]
          tunnel: w355 -> [w364 w366]
          tunnel: [w364 w365] -> w354
          frame "Enabled", Default {
          }
          frame "Disabled and Grayed Out" {
            n165 = for {
              tunnel: w368 -> [w379] mode=indexing
              tunnel: w367 -> [w372]
              shift-right: [w371] -> w365
              shift-left: w366 -> [w370]
              stop <- w373 stop-if-true
              n166 = property class="Ctl"(reference=w379) -> (reference out=w369:refnum<vi>, "Bounds"=w375:T10, "Position"=w374:T12)  [unwired: 1 in, 1 out]
              n167 = Add(x=w375, y=w374) -> (x+y=w378:T10)
              n168 = In Range and Coerce(upper limit=w378, x=w372, lower limit=w374) -> (In Range?=w377:cluster{"Width":bool, "Height":bool})  [unwired: 1 out]
              n169 = Cluster To Array(cluster=w377) -> (array=w376:bool[])
              n170 = And Array Elements(Boolean array=w376) -> (logical AND=w373:bool)
              n171 = case shown="真" w373 {
                tunnel: [w380 w383] -> w371
                tunnel: w370 -> [w380 w383]
                tunnel: w369 -> [_ w389]
                frame False {
                }
                frame True {
                  n172 = Unbundle By Name(w383) -> ("Queue Ref.Data"=w381:refnum<queue>, "Queue Ref.Name"=w382:string)
                  n173 = property class="Ctl"(reference=w389) -> (reference out=w387:refnum<vi>, "Desc"=w388:string)  [unwired: 1 in, 1 out]
                  n174 = call "FlowChart Edit.vi"("Name"=w382, "Identifier In"=w388) -> ("OK？"=w386:bool, "Tips"=w384:string, "Identifier Out"=w385:string)  [unwired: 6 in, 1 out]
                  n175 = case shown="真" w386 {
                    tunnel: w387 -> [_ w394]
                    tunnel: w385 -> [_ w393]
                    tunnel: w384 -> [_ w392]
                    tunnel: w381 -> [_ w391]
                    frame False {
                    }
                    frame True {
                      n176 = property class="Ctl"(reference=w394, "Desc"=w393, "TipStrip"=w392) -> ()  [unwired: 1 in, 2 out]
                      n177 = call "Queue In.vi"("Message"="Flow Chart Save", "Queue In"=w391) -> ()  [unwired: 8 in, 2 out]
                    }
                  }
                }
              }
            }
          }
        }
      }
      frame "Write Prepare" {
        n178 = Unbundle By Name(w405) -> ("Queue Ref.Caller"=w395:refnum<queue>, "Controls"=w404:refnum<vi>[])
        n179 = Variant To Data(type=cluster{i32, "Value":string} {0, "Value"=""}, Variant=w406) -> (data=w407:cluster{i32, "Value":string})  [unwired: 1 in, 1 out]
        n180 = Unbundle(w407) -> (w402:i32, "Value"=w398:string)
        n181 = Index Array(array=w404, index=w402) -> (element=w403:refnum<vi>)
        n182 = Equal?(x=w398, y="1") -> (x = y?=w396:bool)
        n183 = property class="Ctl"(reference=w403) -> ("TipStrip"=w401:string, "Desc"=w400:string)  [unwired: 1 in, 2 out]
        n184 = case shown="\"eee\", 默认" w400 {
          selector: w400 -> [w411 _]
          tunnel: w401 -> [w414 _]
          tunnel: w396 -> [w410 _]
          tunnel: w395 -> [w412 _]
          frame "eee", Default {
            n185 = Select(t="打开", s=w410, f="关闭") -> (s? t:f=w415:string)
            n186 = Format Into String(format string="确定%s%s?" ("消息"), w415, w414) -> (resulting string=w418:string)  [unwired: 2 in, 1 out]
            n187 = Two Button Dialog(message=w418) -> (T button?=w413:bool)  [unwired: 2 in]
            n188 = case shown="真" w413 {
              tunnel: w412 -> [_ w423]
              tunnel: w411 -> [_ w422]
              tunnel: w410 -> [_ w421]
              frame False {
              }
              frame True {
                n189 = call "000_Bool True.vi"("Value"=w421) -> ("String Out"=w420:string)  [unwired: 8 in, 2 out]
                n190 = call "000_Source Write.vim"("Data"=w420, "Name"=w422, "Queue In"=w423) -> ()  [unwired: 6 in, 3 out]
              }
            }
          }
          frame "" {
          }
        }
      }
      frame "ShowLable" {
        n191 = Unbundle By Name(w426) -> ("Controls"=w425:refnum<vi>[])
        n192 = for {
          tunnel: w425 -> [w430] mode=indexing
          tunnel: "ShowLable" -> [w429]
          n193 = property class="Ctl"(reference=w430, "Caption.Visible"=w429) -> ()  [unwired: 1 in, 2 out]
        }
      }
      frame "Exit" {
        n194 = Unbundle By Name(w432) -> ("Queue Ref.UE"=w431:refnum<user-event>, "Queue Ref.Message"=w436:refnum<queue>, "Queue Ref.Data"=w435:refnum<queue>)
        n195 = Build Array(w436, w435) -> (w434:refnum<queue>[])
        n196 = for {
          tunnel: w434 -> [w444] mode=indexing
          tunnel: w433 -> [w443]
          n197 = call "Queue In.vi"("First"=TRUE, "Message"=w443, "Queue In"=w444) -> ()  [unwired: 7 in, 2 out]
        }
        n198 = Generate User Event(user event=w431, event data cluster=w433) -> ()  [unwired: 2 in, 2 out]
        n199 = call "Queue Clear.vi"("error in (no error)"=w438, "Queue In"=w440) -> ("error out"=w437:errorcluster, "Queue Out"=w439:refnum<queue>)  [unwired: 8 in]
      }
      frame "Quit" {
      }
    }
    n200 = call "Queue In.vi"("error in (no error)"=w274, "Message"=w273, "Queue In"=w277) -> ("error out"=w275:errorcluster, "Queue Out"=w276:refnum<queue>)  [unwired: 7 in]
  }
  n201 = call "000 Driver Message.vi"("Queue In"=w3) -> ("error out"=w42:errorcluster)  [unwired: 8 in, 2 out]
  n202 = call "Queue Release.vi"("error in (no error)"=w40, "Queue In"=w39) -> ("error out"=w43:errorcluster)  [unwired: 9 in]
  n203 = call "Queue Release.vi"("error in (no error)"=w32, "Queue In"=w31) -> ("error out"=w35:errorcluster)  [unwired: 9 in]
  n204 = Unregister For Events(event registration refnum=w29) -> (error out=w30:errorcluster)  [unwired: 1 in]
  n205 = Destroy User Event(user event=w2, error in=w30) -> (error out=w34:errorcluster)
  n206 = Call Chain() -> (call chain=w37:string[])
  n207 = Merge Errors(w34, w35, w42, w43) -> (w36:errorcluster)
  n208 = Array Size(array=w37) -> (size(s)=w38:i32)
  n209 = case shown="2.." w38 {
    tunnel: w36 -> [_ w449]
    frame 0, Default {
    }
    frame 2.. {
      n210 = invoke class="VI" method="FP.Close"(error in=w449) -> ()  [unwired: 2 in, 3 out]
    }
  }
